vi "Get String.vi"(8 "error in (no error)":errorcluster, 11 "StringMsg in":refnum<class "StringMessage.lvclass">) -> (0 "error out":errorcluster, 2 "Message Data":string, 3 "StringMsg out":refnum<class "StringMessage.lvclass">)   [LabVIEW 2009, in "LapDog.Messaging.v2.NativeTypes.lvlib" / "StringMessage.lvclass"]
doc: "Returns the data contained in the message.\n\nThis method executes regardless of the error in state."
uses:
  StringMessage.lvclass
  StringMessage.lvclass/StringMessage.ctl
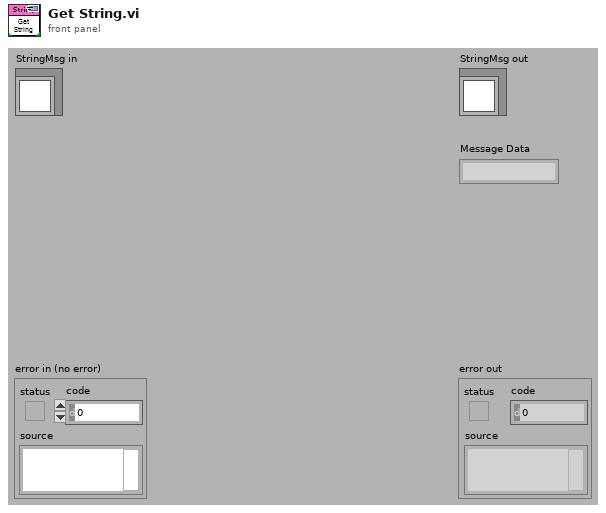
[diagram p1: front panel]
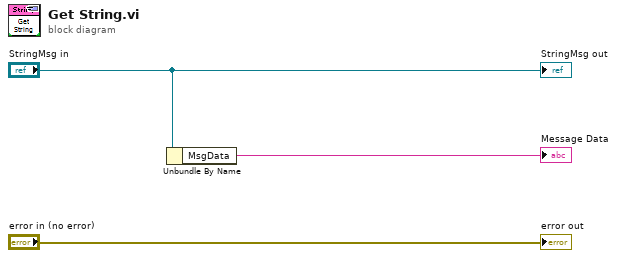
[diagram p0: block diagram]
diagram:
  n1 = Unbundle By Name("StringMsg in") -> ("MsgData"=→"Message Data":string)
  "error out" <- "error in (no error)"
  "StringMsg out" <- "StringMsg in"
